vi "Test.vi"() -> ()   [LabVIEW 2020]
uses:
  Classes/Topic/Topic.lvclass
  Classes/TOC/TOC.lvclass
panel:
  out "XML String":string
  out "XML":string
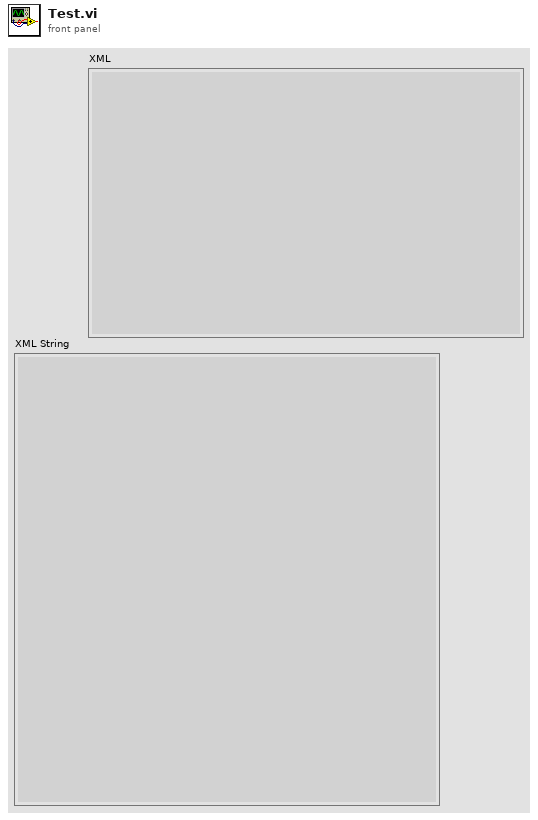
[diagram p1: front panel]
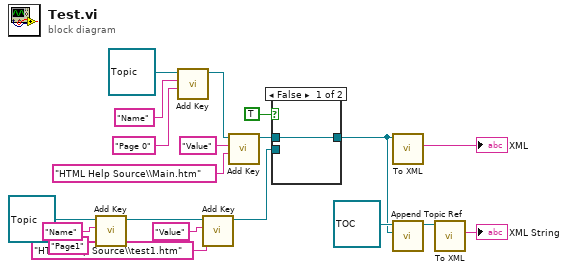
[diagram p0: block diagram]
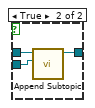
[diagram p2: hidden frame]
diagram:
  n1 = call-dynamic "Add Key.vi"("value"="Page1", "name"="Name", "Topic in"=refnum<class "Topic.lvclass"> refnum) -> ("Topic out"=w15:refnum<class "Topic.lvclass">)  [unwired: 6 in, 2 out]
  n2 = call-dynamic "Add Key.vi"("value"="Page 0", "name"="Name", "Topic in"=refnum<class "Topic.lvclass"> refnum) -> ("Topic out"=w17:refnum<class "Topic.lvclass">)  [unwired: 6 in, 2 out]
  n3 = call-dynamic "Add Key.vi"("value"="HTML Help Source\\test1.htm", "name"="Value", "Topic in"=w15) -> ("Topic out"=w11:refnum<class "Topic.lvclass">)  [unwired: 6 in, 2 out]
  n4 = call-dynamic "Add Key.vi"("value"="HTML Help Source\\Main.htm", "name"="Value", "Topic in"=w17) -> ("Topic out"=w16:refnum<class "Topic.lvclass">)  [unwired: 6 in, 2 out]
  n5 = case shown="False" TRUE {
    tunnel: w16 -> [w21 w24]
    tunnel: w11 -> [_ w23]
    tunnel: [w21 w22] -> w8
    frame False {
    }
    frame True {
      n6 = call-dynamic "Append Subtopic.vi"("SubTopic In"=w23, "Topic in"=w24) -> ("Topic out"=w22:refnum<class "Topic.lvclass">)  [unwired: 8 in, 1 out]
    }
  }
  n7 = call-dynamic "To XML.vi"("Topic in"=w8) -> ("XML String"=→"XML":string)  [unwired: 8 in, 2 out]
  n8 = call-dynamic "Append Topic Ref.vi"("Topic In"=w8, "TOC in"=refnum<class "TOC.lvclass"> refnum ("TOC.lvclass")) -> ("TOC out"=w7:refnum<class "TOC.lvclass">)  [unwired: 8 in, 1 out]
  n9 = call-dynamic "To XML.vi"("TOC in"=w7) -> ("XML String"=→"XML String":string)  [unwired: 8 in, 2 out]
